vi "Transmit.vi"(7 "packet? (f)":bool, 8 "error in (no error)":errorcluster, 10 "Data":string, 11 "Socket.UDP in":refnum<class "Socket.UDP.lvclass">) -> (0 "error out":errorcluster, 2 "bytes sent":i32, 3 "Socket.UDP out":refnum<class "Socket.UDP.lvclass">)   [LabVIEW 2014, in "Socket.lvlib" / "Socket.UDP.lvclass"]
doc: "Transmits the data, returns the number of bytes transmitted\n\n string data: Data to be transmitted.\n\nbool packet? : Ignored for UDP."
uses:
  Socket.UDP.lvclass
  Socket.UDP.lvclass/Socket.UDP.ctl
  Socket.Base/Socket.Base.lvclass/Socket.Base.ctl
  Accessors/Read remote_port .vi
  Accessors/Read remote_address .vi
  Accessors/Read udp_refnum.vi
  Socket.Base/Accessors/Read timeout.vi
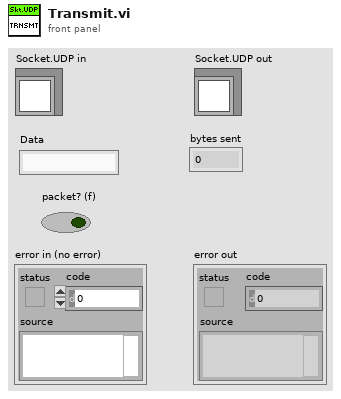
[diagram p1: front panel]
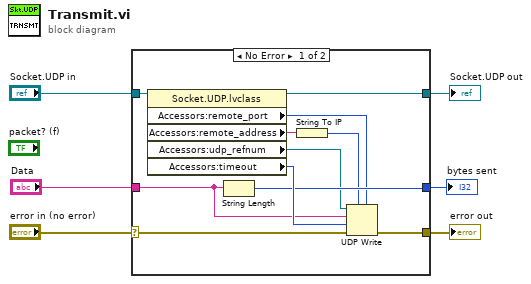
[diagram p0: block diagram]
diagram:
  n1 = case shown="No Error" "error in (no error)" {
    selector: "error in (no error)" -> [w16 w19]
    tunnel: [w14 w19] -> w5
    tunnel: [w15 w18] -> w3
    tunnel: "Socket.UDP in" -> [w17 w18]
    tunnel: "Data" -> [w12 _]
    tunnel: [w11 _] -> w1
    frame No Error {
      n2 = property class="Socket.UDP.lvclass"(reference=w17) -> (reference out=w15:refnum<class "Socket.UDP.lvclass">, "Accessors:remote_port "=w8:u16, "Accessors:remote_address "=w10:string, "Accessors:udp_refnum"=w7:refnum<k16>, "Accessors:timeout"=w13:i32)  [unwired: 1 in, 1 out]
      n3 = String Length(string=w12) -> (length=w11:i32)
      n4 = String To IP(1:w10) -> (0:w9:u32)
      n5 = UDP Write(address=w9, port or service name=w8, connection ID=w7, data in=w12, 8:w16, 9:w13) -> (error out=w14:errorcluster)  [unwired: 1 out]
    }
    frame Error {
    }
  }
  "error out" <- w5
  "Socket.UDP out" <- w3
  "bytes sent" <- w1
